vi "READ_KEITHLEY2470.vi"(8 "error in (no error)":errorcluster, 11 "VISA resource name":refnum<visa-resource-name>) -> (0 "error out":errorcluster, 2 "DATA":dbl[](array[numeric]), 3 "VISA resource name out":refnum<visa-resource-name>)   [LabVIEW 2019]
uses:
  <instrlib>/Keithley 2450/Keithley 2450.lvlib
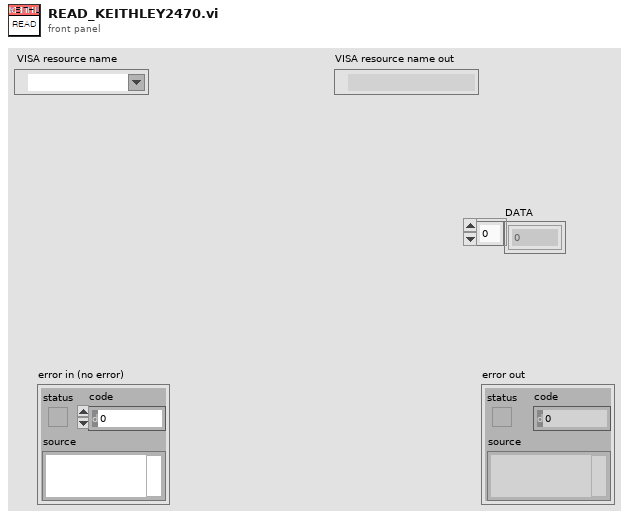
[diagram p1: front panel]
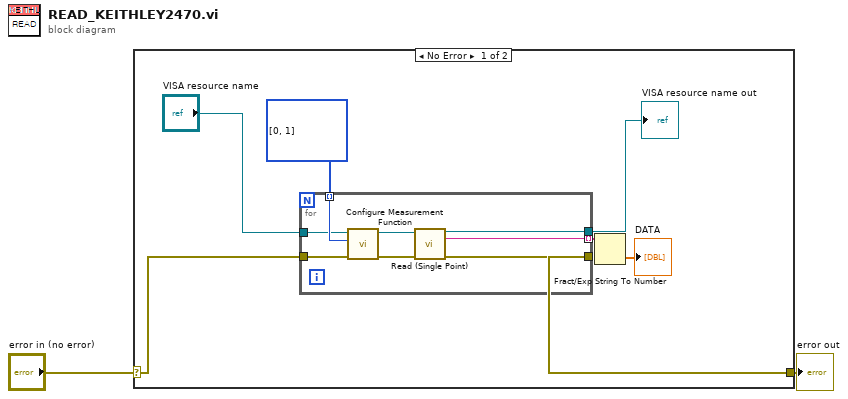
[diagram p0: block diagram]
diagram:
  n1 = case shown="No Error" "error in (no error)" {
    selector: "error in (no error)" -> [w7 w18]
    tunnel: [w6 w18] -> w1
    frame No Error {
      w8 = u16[] [0, 1] items=["Volts", "Current", "Auto Resistance"]
      n2 = for {
        tunnel: [w17] -> w9 mode=indexing
        tunnel: [w16] -> w6
        tunnel: w8 -> [w15] mode=indexing
        tunnel: w7 -> [w12]
        tunnel: [w11] -> w4
        tunnel: "VISA resource name" -> [w10]
        n3 = call <instrlib>:"Configure Measurement Function.vi"("error in (no error)"=w12, "Function (0: Volts)"=w15, "VISA resource name"=w10) -> ("error out"=w13:errorcluster, "VISA resource name out"=w14:refnum<visa-resource-name>)  [unwired: 7 in]
        n4 = call <instrlib>:"Read (Single Point).vi"("VISA resource name"=w14, "error in (no error)"=w13) -> ("VISA resource name out"=w11:refnum<visa-resource-name>, "Data out"=w17:string, "error out"=w16:errorcluster)  [unwired: 11 in]
      }
      "VISA resource name out" <- w4
      n5 = Fract/Exp String To Number(string=w9) -> (number=→"DATA":dbl[])  [unwired: 3 in, 1 out]
    }
    frame Error {
    }
  }
  "error out" <- w1
